vi "Close Connection with CD.vi"(8 "error in (no error)":errorcluster, 11 "connection info":T1) -> (0 "error out":errorcluster)   [LabVIEW 2019, in "J1939 Host Automation API.lvlib"]
uses:
  J1939 Host Automation API.lvlib
  Addon/Addon Shared/J1939 Addon Shared.lvlib
  <vilib>/NI/STM/SubVIs/MetaDataElement.ctl
  <vilib>/NI/STM/NI STM.lvlib
  <vilib>/NI/STM/TCP/TCP Connection Info.ctl
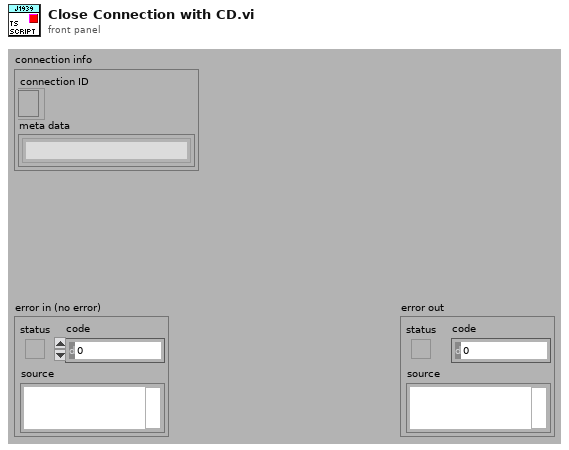
[diagram p1: front panel]
types:
  T1 = typedef "NI STM.lvlib/TCP Connection Info.ctl" = cluster{"connection ID":refnum<k5>, "meta data":T2[]}
  T2 = typedef "NI STM.lvlib/MetaDataElement.ctl" = string
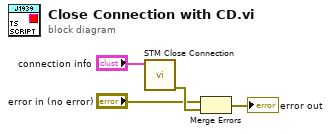
[diagram p0: block diagram]
diagram:
  n1 = call "STM Close Connection.vi"("connection info"="connection info") -> ("error out"=w4:errorcluster)  [unwired: 10 in]
  n2 = Merge Errors("error in (no error)", w4) -> (→"error out":errorcluster)
